vi "Reading and Writing Data with an Offset.vi"() -> ()   [LabVIEW 2012]
uses:
  User Controls/Array Dimensions.ctl
  User Controls/Offset.ctl
  Non-User VIs/Allocate Memory/AllocateMemory_u32.vi
  Non-User VIs/Write Memory/WriteMemory_u32.vi
  Non-User VIs/Read Memory/ReadMemory 32u .vi
  Non-User VIs/Error Checking/View Error Log Mode Functional Global.vi
  OpenCLV x64.lvlib
panel:
  out "All Data":dbl[][][](array[numeric])
  out "2nd Element":dbl[][][](array[numeric])
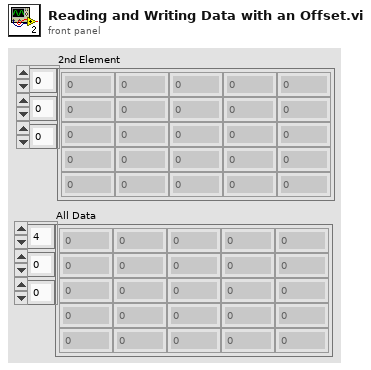
[diagram p1: front panel]
types:
  T1 = typedef "Offset.ctl" = cluster{"X":u64, "Y":u64, "Z":u64}
  T2 = typedef "Array Dimensions.ctl" = cluster{"Depth":u64, "Height":u64, "Width":u64}
  T3 = typedef "OpenCLV x64.lvlib/Device ID.ctl" = u64
  T4 = typedef "OpenCLV x64.lvlib/Memory Object.ctl" = cluster{"Device ID":T3, "Memeroy ID":T5, "Dimension":T2, "Memory Type":T6}
  T5 = typedef "OpenCLV x64.lvlib/Memory ID.ctl" = u64
  T6 = typedef "OpenCLV x64.lvlib/Memory Type.ctl" = enum16{"32f", "u8", "i8", "u16", "i16", "u32", "i32", "64f"}
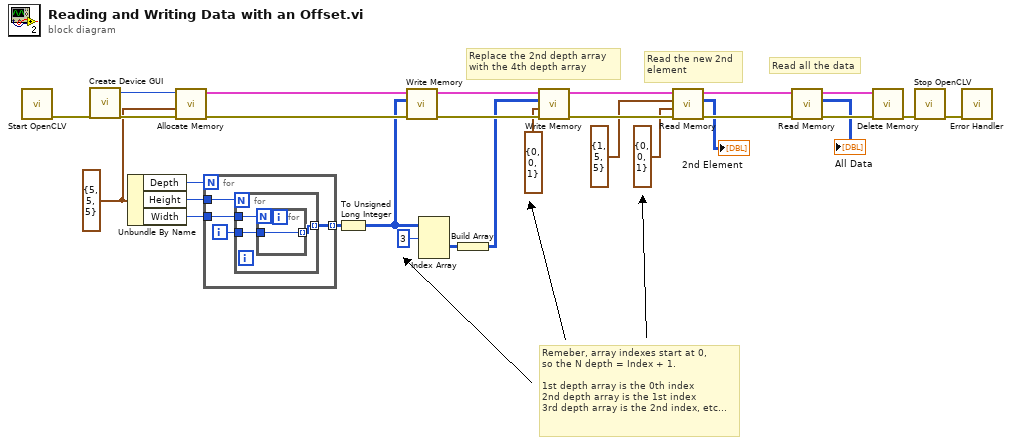
[diagram p0: block diagram]
diagram:
  w15 = T2 {"Depth"=5, "Height"=5, "Width"=5} ("Dimension")
  # "Remeber, array indexes start at 0,\nso the N depth = Index + 1.\n\n1st depth array is the 0th index\n2nd depth array is the 1st index\n3rd depth array is the 2nd index, etc..."
  # "Read all the data"
  # "Read the new 2nd\nelement"
  # "Replace the 2nd depth array \nwith the 4th depth array"
  n1 = call "Start OpenCLV.vi"() -> ("Error Out"=w29:errorcluster)  [unwired: 11 in]
  n2 = call "Create Device GUI.vi"("Error In"=w29) -> ("error constant"=w28:errorcluster, "Device Reference"=w27:T3)  [unwired: 9 in]
  n3 = Unbundle By Name(w15) -> ("Depth"=w26:u64, "Height"=w25:u64, "Width"=w9:u64)
  n4 = call-poly "Allocate Memory.vi"("Error In"=w28, "Dimension"=w15, "Device In"=w27) -> ("Error Out"=w23:errorcluster, "Memory Object"=w24:T4)  [unwired: 6 in, 1 out]
  n5 = for {
    N: w26 -> [_]
    tunnel: w25 -> [w33]
    tunnel: [w31] -> w8 mode=indexing
    tunnel: w9 -> [w30]
    i -> [w32]
    n6 = for {
      N: w33 -> [_]
      tunnel: w32 -> [w36]
      tunnel: [w35] -> w31 mode=indexing
      tunnel: w30 -> [w34]
      n7 = for {
        N: w34 -> [_]
        tunnel: w36 -> [w37]
        tunnel: [w37] -> w35 mode=indexing
      }
    }
  }
  n8 = To Unsigned Long Integer(number=w8) -> (unsigned 32bit integer=w1:u32[][][])
  n9 = call-poly "Write Memory.vi"("Error In"=w23, "Data In"=w1, "Memory Object In"=w24) -> ("Error Out"=w22:errorcluster, "Memory Object Out"=w21:T4)  [unwired: 6 in, 1 out]
  n10 = Index Array(array=w1, index (dim 0)=3 ("index (page)")) -> (element=w19:u32[][])  [unwired: 2 in]
  n11 = Build Array(w19) -> (w18:u32[][][])
  n12 = call-poly "Write Memory.vi"("Error In"=w22, "Offset"=T1 {"X"=0, "Y"=0, "Z"=1}, "Data In"=w18, "Memory Object In"=w21) -> ("Error Out"=w5:errorcluster, "Memory Object Out"=w6:T4)  [unwired: 5 in, 1 out]
  n13 = call-poly "Read Memory.vi"("Error In"=w5, "Offset"=T1 {"X"=0, "Y"=0, "Z"=1}, "Dimensions"=T2 {"Depth"=1, "Height"=5, "Width"=5}, "Memory Object In"=w6) -> ("Error Out"=w16:errorcluster, "Data Out"=→"2nd Element":u32[][][], "Memory Object Out"=w17:T4)  [unwired: 4 in, 1 out]
  n14 = call-poly "Read Memory.vi"("Error In"=w16, "Memory Object In"=w17) -> ("Error Out"=w13:errorcluster, "Data Out"=→"All Data":u32[][][], "Memory Object Out"=w14:T4)  [unwired: 6 in, 1 out]
  n15 = call "Delete Memory.vi"("Error In"=w13, "Memory Object In"=w14) -> ("Error Out"=w12:errorcluster)  [unwired: 8 in, 1 out]
  n16 = call "Stop OpenCLV.vi"("Error In"=w12) -> ("Error Out"=w11:errorcluster)  [unwired: 10 in]
  n17 = call-poly "Error Handler.vi"("Error In"=w11) -> ()  [unwired: 10 in, 1 out]
